vi "Write IDs.vi"(8 "error in (no error)":errorcluster, 10 "IDs":string[](array[string]), 11 "PPT in":refnum<class "PPT.lvclass">) -> (0 "error out":errorcluster, 3 "PPT out":refnum<class "PPT.lvclass">)   [LabVIEW 2014]
uses:
  PPT.lvclass
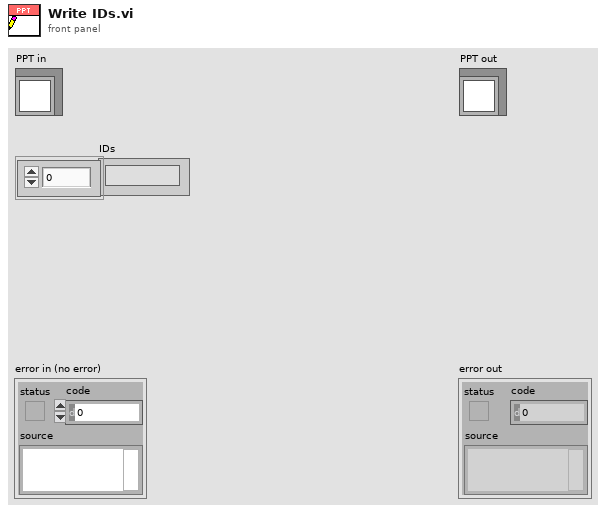
[diagram p1: front panel]
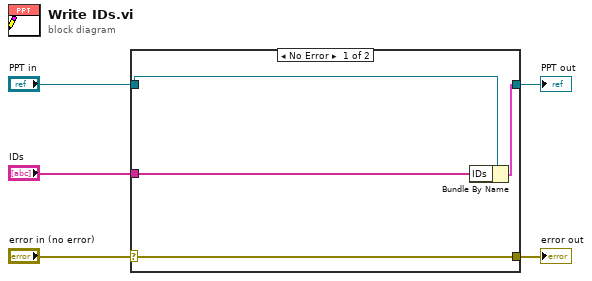
[diagram p0: block diagram]
diagram:
  n1 = case shown="No Error" "error in (no error)" {
    selector: "error in (no error)" -> [w9 w10]
    tunnel: [w9 w10] -> w4
    tunnel: [w7 w11] -> w2
    tunnel: "PPT in" -> [w8 w11]
    tunnel: "IDs" -> [w6 _]
    frame No Error {
      n2 = Bundle By Name(cluster=w8, "IDs"=w6) -> (w7:cluster{})
    }
    frame Error {
    }
  }
  "error out" <- w4
  "PPT out" <- w2
